vi "PrepDitheredImageNamesForPrintingGeneric.vi"(6 "HeadUsed":bool, 8 "error in (no error)":errorcluster, 9 "String":string, 10 "Head":i32, 11 "PPP_Dithered_Images":path) -> (0 "error out":errorcluster, 2 "new path":path, 3 "appended path":path)   [LabVIEW 2022 SP3, in "TopLevel.lvclass"]
uses:
  TopLevel.lvclass
  Common/Controls/DLPConfig)Init_HeadPropertyAttr--Cluster.ctl
  DLP2/DataTypes/DLP2_PrinterHeadProperties.ctl
  DLP2/DataTypes/DLP2_PrinterMaterialProperties.ctl
  Common/Controls/DLP_MaterialToHeadMapping--Cluster.ctl
panel:
  in  "TopLevel.lvclass":refnum<class "TopLevel.lvclass">
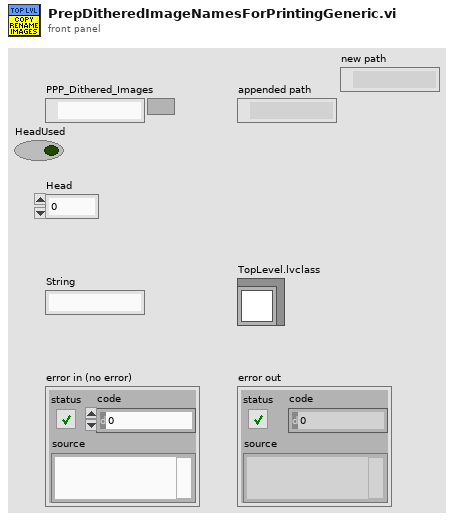
[diagram p1: front panel]
types:
  T1 = typedef "DLP2_PrinterHeadProperties.ctl" = cluster{"#attributes":T2}
  T2 = typedef "DLPConfig)Init_HeadPropertyAttr--Cluster.ctl" = cluster{"HeadNumber":u8, "Material":string, "HeadLocalX":dbl, "HeadLocalY":dbl, "HeadRotationAngle":dbl, "VH2L_Hi":dbl, "VH2R_Hi":dbl, "VH1LA_Hi":dbl, "VH1LB_Hi":dbl, "VH1RA_Hi":dbl, "VH1RB_Hi":dbl, "VH2L_Lo":dbl, "VH2R_Lo":dbl, "VH1LA_Lo":dbl, "VH1LB_Lo":dbl, "VH1RA_Lo":dbl, "VH1RB_Lo":dbl}
  T3 = typedef "TD Dynamic CVT DVR--ref.ctl" = refnum<data-value>
  T4 = typedef "DLP_MaterialToHeadMapping--Cluster.ctl" = cluster{"Head":u8, "Ink":T5}
  T5 = typedef "DLP2_PrinterMaterialProperties.ctl" = cluster{"#attributes":cluster{"InkType":string, "PrePrintPurge":bool, "PurgeTime":dbl, "PurgeCount":i32, "Density":dbl, "NumberofDrops":i32, "PrintWeight":dbl, "PrintheadPrime":bool}, "Idle":cluster{"Name":string, "Heat":dbl, "Meniscus":dbl, "Recirculation":bool}[], "Process":cluster{"Name":string, "Heat":dbl, "Meniscus":dbl, "Recirculation":bool, "ColorPlane":string}[]}
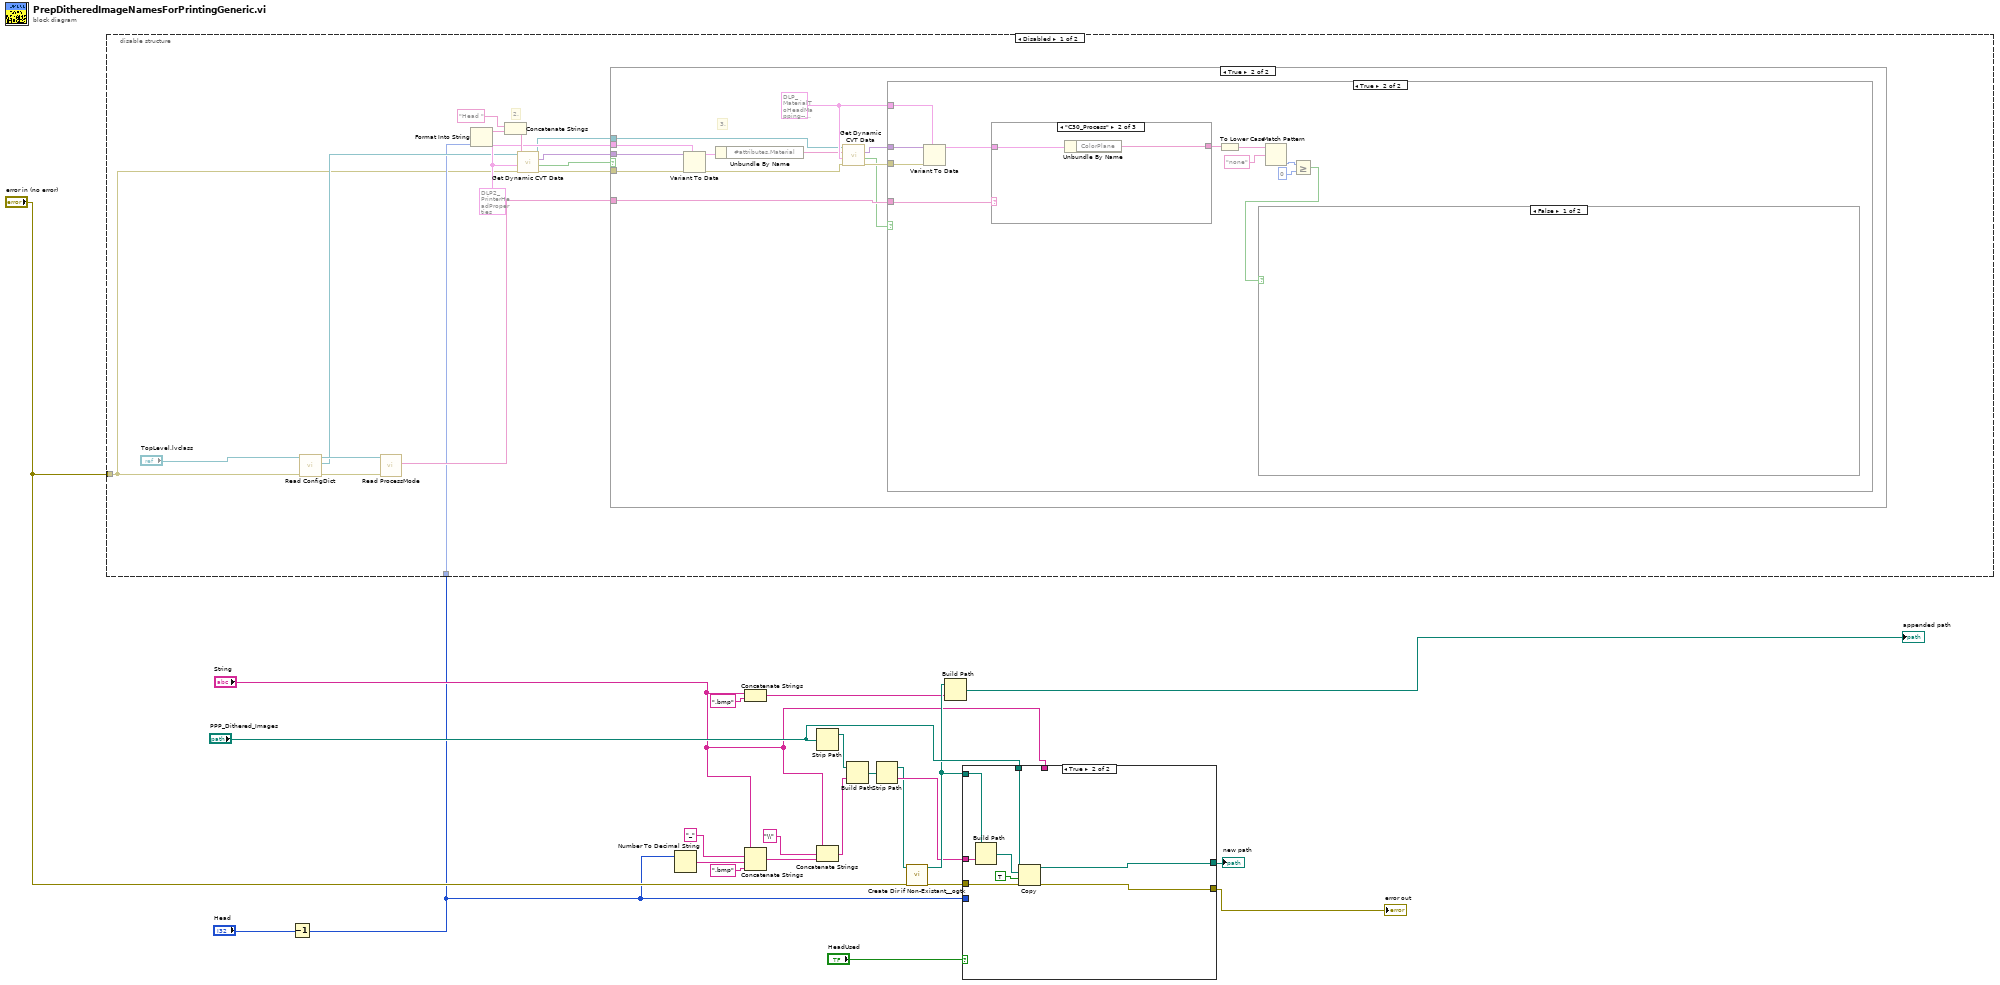
[diagram p0: block diagram]
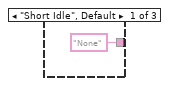
[diagram p5: hidden frame]
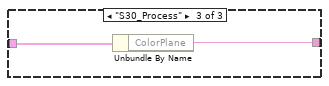
[diagram p6: hidden frame]
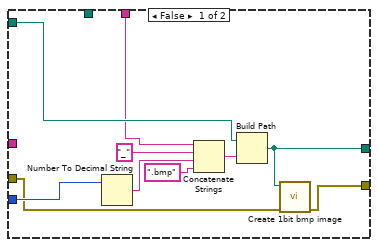
[diagram p8: hidden frame]
diagram:
  n1 = Decrement(x="Head") -> (x-1=w1:i32)
  n2 = disable-structure shown="Disabled" {
    disable-tunnel: w1 -> [w25 _]
    disable-tunnel: "error in (no error)" -> [w24 _]
    frame Disabled {
      w33 = T1 {"#attributes"={"HeadNumber"=0, "Material"="", "HeadLocalX"=0.0, "HeadLocalY"=0.0, "HeadRotationAngle"=0.0, "VH2L_Hi"=0.0, "VH2R_Hi"=0.0, "VH1LA_Hi"=0.0, "VH1LB_Hi"=0.0, "VH1RA_Hi"=0.0, "VH1RB_Hi"=0.0, "VH2L_Lo"=0.0, "VH2R_Lo"=0.0, "VH1LA_Lo"=0.0, "VH1LB_Lo"=0.0, "VH1RA_Lo"=0.0, "VH1RB_Lo"=0.0}}
      # "2."
      n3 = call-dynamic "Read ConfigDict.vi"("error in (no error)"=w24, "TopLevel in"="TopLevel.lvclass") -> ("error out"=w27:errorcluster, "ConfigDIct"=w28:T3, "TopLevel out"=w29:refnum<class "TopLevel.lvclass">)  [unwired: 7 in]
      n4 = call-dynamic "Read ProcessMode.vi"("error in (no error)"=w27, "TopLevel in"=w29) -> ("ProcessMode"=w26:string)  [unwired: 7 in, 2 out]
      n5 = Format Into String(w25) -> (resulting string=w37:string)  [unwired: 3 in, 1 out]
      n6 = Concatenate Strings("Head " ("string"), w37) -> (w34:string)
      n7 = call <vilib>:"Get Dynamic CVT Data.vi"("error in (no error)"=w24, "default value (empty variant)"=w33, "DataName"=w34, "dCVT DVR"=w28) -> ("error out"=w35:errorcluster, "found"=w32:bool, "value"=w36:variant, "dCVT DVR out"=w31:T3)  [unwired: 4 in]
      n8 = case shown="True" w32 {
        tunnel: w36 -> [_ w50]
        tunnel: w35 -> [_ w49]
        tunnel: w33 -> [_ w48]
        tunnel: w31 -> [_ w41]
        tunnel: w26 -> [_ w40]
        frame False {
        }
        frame True {
          w44 = T4 {"Head"=0, "Ink"={"#attributes"={"InkType"="", "PrePrintPurge"=FALSE, "PurgeTime"=0.0, "PurgeCount"=0, "Density"=0.0, "NumberofDrops"=0, "PrintWeight"=0.0, "PrintheadPrime"=FALSE}, "Idle"=[], "Process"=[]}}
          # "3."
          n9 = Variant To Data(error in=w49, type=w48, Variant=w50) -> (data=w47:T1, error out=w42:errorcluster)
          n10 = Unbundle By Name(w47) -> ("#attributes.Material"=w43:string)
          n11 = call <vilib>:"Get Dynamic CVT Data.vi"("error in (no error)"=w42, "default value (empty variant)"=w44, "DataName"=w43, "dCVT DVR"=w41) -> ("error out"=w46:errorcluster, "found"=w39:bool, "value"=w45:variant)  [unwired: 4 in, 1 out]
          n12 = case shown="True" w39 {
            tunnel: w46 -> [_ w61]
            tunnel: w45 -> [_ w60]
            tunnel: w44 -> [_ w59]
            tunnel: w40 -> [_ w57]
            frame False {
            }
            frame True {
              n13 = Variant To Data(error in=w61, type=w59, Variant=w60) -> (data=w58:T4)  [unwired: 1 out]
              n14 = case shown="\"C30_Process\"" w57 {
                tunnel: w58 -> [_ w64 w66]
                tunnel: ["None" ("ColorPlane") w63 w65] -> w56
                frame "Short Idle", Default {
                }
                frame "C30_Process" {
                  n15 = Unbundle By Name(w64) -> ("ColorPlane"=w63:string)
                }
                frame "S30_Process" {
                  n16 = Unbundle By Name(w66) -> ("ColorPlane"=w65:string)
                }
              }
              n17 = To Lower Case(string=w56) -> (all lower case string=w55:string)
              n18 = Match Pattern(string=w55, regular expression="none") -> (offset past match=w53:i32)  [unwired: 1 in, 3 out]
              n19 = Greater Or Equal?(x=w53, y=0) -> (x >= y?=w51:bool)
              n20 = case shown="False" w51 {
                frame False {
                }
                frame True {
                }
              }
            }
          }
        }
      }
    }
    frame Enabled {
    }
  }
  n21 = Number To Decimal String(number=w1) -> (decimal integer string=w12:string)  [unwired: 1 in]
  n22 = Concatenate Strings("String", ".bmp" ("string")) -> (w20:string)
  n23 = Concatenate Strings("String", "_" ("string"), w12, ".bmp" ("string")) -> (w14:string)
  n24 = Strip Path(path="PPP_Dithered_Images") -> (stripped path=w8:path)  [unwired: 1 out]
  n25 = Concatenate Strings("String", "\\" ("string"), w14) -> (w10:string)
  n26 = Build Path(base path=w8, name or relative path=w10) -> (appended path=w17:path)
  n27 = Strip Path(path=w17) -> (stripped path=w18:path, name=w19:string)
  n28 = call <userlib>:"Create Dir if Non-Existant__ogtk.vi"("error in (no error)"="error in (no error)", "Directory Path"=w18) -> ("error out"=w15:errorcluster, "dup Directory Path"=w22:path)  [unwired: 7 in, 1 out]
  n29 = Build Path(base path=w22, name or relative path=w20) -> (appended path=→"appended path":path)
  n30 = case shown="True" "HeadUsed" {
    tunnel: "PPP_Dithered_Images" -> [_ w84]
    tunnel: [w69 w83] -> w4
    tunnel: w22 -> [w72 w82]
    tunnel: w19 -> [_ w80]
    tunnel: w15 -> [w68 w79]
    tunnel: "String" -> [w71 _]
    tunnel: w1 -> [w70 _]
    tunnel: [w67 w77] -> w2
    frame False {
      n31 = Number To Decimal String(number=w70) -> (decimal integer string=w74:string)  [unwired: 1 in]
      n32 = Concatenate Strings(w71, "_" ("string"), w74, ".bmp" ("string")) -> (w76:string)
      n33 = Build Path(base path=w72, name or relative path=w76) -> (appended path=w67:path)
      n34 = call "Create 1bit bmp image.vi"("error in (no error)"=w68, "path to BMP file"=w67) -> ("error out"=w69:errorcluster)  [unwired: 9 in]
    }
    frame True {
      n35 = Build Path(base path=w82, name or relative path=w80) -> (appended path=w81:path)
      n36 = Copy(8:w79, 9:TRUE ("overwrite (F)"), 10:w81, 11:w84) -> (0:w83:errorcluster, 3:w77:path)  [unwired: 1 in, 1 out]
    }
  }
  "error out" <- w4
  "new path" <- w2
